vi "Dashboard.vi"   [LabVIEW 2019]
uses:
  <vilib>/Rock Robotics/Network Tables/NT Read Boolean.vi
  <vilib>/Rock Robotics/Network Tables/NT Write Number.vi
  Drive Global.vi
  <vilib>/Rock Robotics/Network Tables/NT Read Number.vi
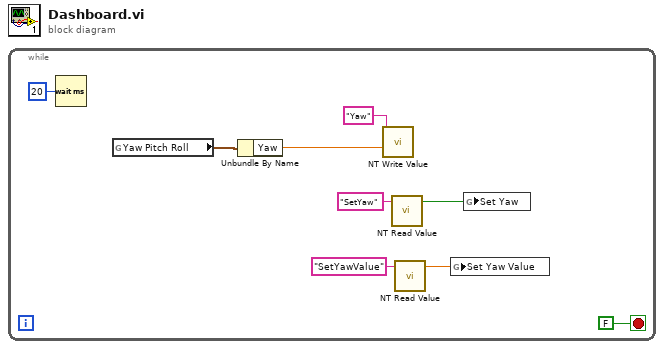
[diagram p0: block diagram]
diagram:
  n1 = while {
    stop <- FALSE stop-if-true
    n2 = Wait (ms)(milliseconds to wait=u32 20) -> ()  [unwired: 1 out]
    n3 = global read "Drive Global.vi" "Yaw Pitch Roll"() -> (w5:cluster{"Yaw":dbl, "Pitch":dbl, "Roll":dbl})
    n4 = Unbundle By Name(w5) -> ("Yaw"=w6:dbl)
    n5 = call-poly <vilib>:"NT Write Value.vi"("Numeric"=w6, "Name"="Yaw") -> ()  [unwired: 9 in, 1 out]
    n6 = call-poly <vilib>:"NT Read Value.vi"("Name"="SetYaw") -> ("Boolean"=w3:bool)  [unwired: 9 in, 1 out]
    n7 = call-poly <vilib>:"NT Read Value.vi"("Name"="SetYawValue") -> ("Numeric"=w2:dbl)  [unwired: 9 in, 1 out]
    n8 = global write "Drive Global.vi" "Set Yaw Value"(w2) -> ()
    n9 = global write "Drive Global.vi" "Set Yaw"(w3) -> ()
  }
